vi "Andres  Decoder 3-to-4 while-loop (why run only once).vi"() -> ()   [LabVIEW 2013]
panel:
  out "Boolean 4":bool
  out "Boolean 3":bool
  out "Boolean 2":bool
  out "Boolean 1":bool
  out "Boolean 0":bool
  in  "Digital 2":bool
  in  "Digital 0":bool
  in  "Digital 1":bool
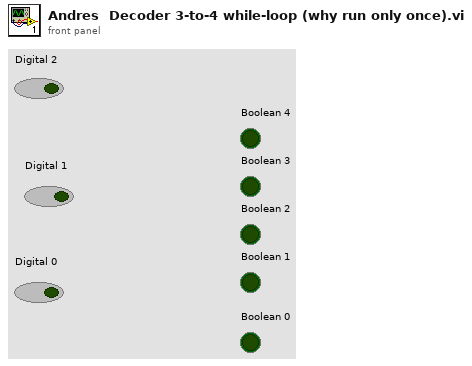
[diagram p1: front panel]
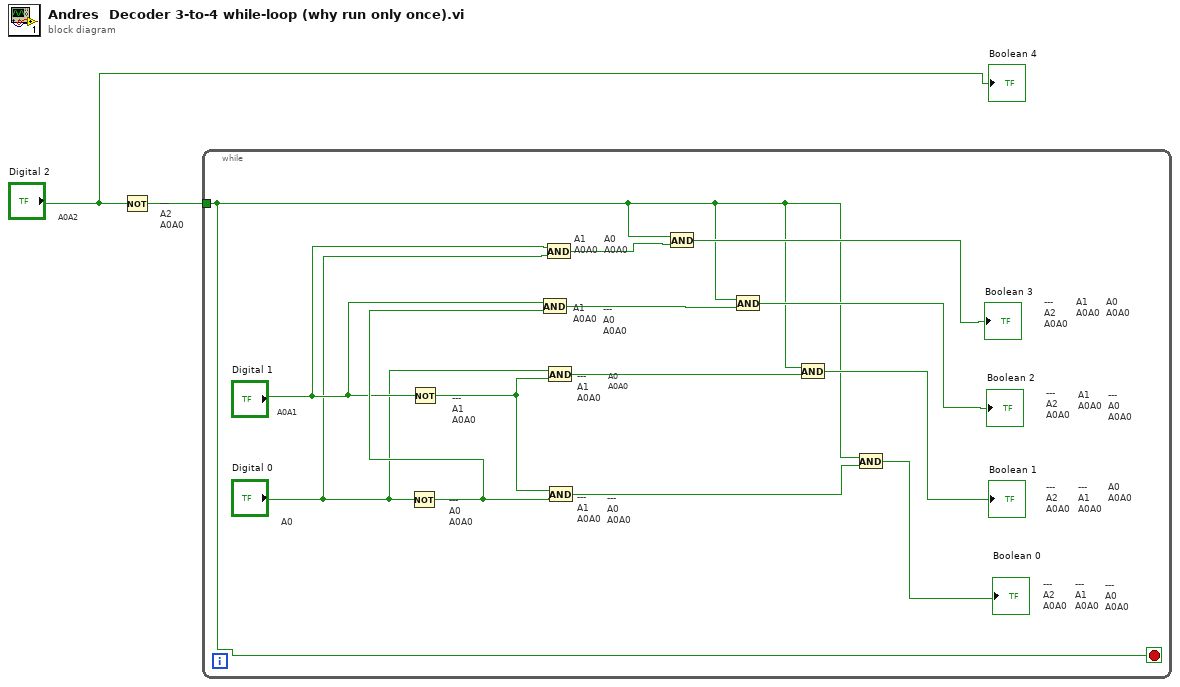
[diagram p0: block diagram]
diagram:
  # "---\nA2\nA0A0"
  # "A0A2"
  n1 = Not(x="Digital 2") -> (.not. x?=w2:bool)
  n2 = while {
    tunnel: w2 -> [w3]
    stop <- w3 stop-if-true
    # "A1\nA0A0"
    # "A0\nA0A0"
    # "---\nA2\nA0A0"
    # "A1\nA0A0"
    # "A0\nA0A0"
    # "A1\nA0A0"
    # "---\nA0\nA0A0"
    # "---\nA2\nA0A0"
    # "A1\nA0A0"
    # "---\nA0\nA0A0"
    # "---\nA1\nA0A0"
    # "A0\nA0A0"
    # "---\nA2\nA0A0"
    # "---\nA1\nA0A0"
    # "A0\nA0A0"
    # "---\nA2\nA0A0"
    # "---\nA1\nA0A0"
    # "---\nA0\nA0A0"
    # "---\nA1\nA0A0"
    # "---\nA0\nA0A0"
    # "---\nA1\nA0A0"
    # "A0A1"
    # "---\nA0\nA0A0"
    # "A0"
    n3 = Not(x="Digital 0") -> (.not. x?=w10:bool)
    n4 = Not(x="Digital 1") -> (.not. x?=w13:bool)
    n5 = And(x="Digital 1", y=w10) -> (x .and. y?=w9:bool)
    n6 = And(x="Digital 1", y="Digital 0") -> (x .and. y?=w5:bool)
    n7 = And(x="Digital 0", y=w13) -> (x .and. y?=w12:bool)
    n8 = And(x=w13, y=w10) -> (x .and. y?=w15:bool)
    n9 = And(x=w3, y=w5) -> (x .and. y?=→"Boolean 3":bool)
    n10 = And(x=w3, y=w9) -> (x .and. y?=→"Boolean 2":bool)
    n11 = And(x=w3, y=w12) -> (x .and. y?=→"Boolean 1":bool)
    n12 = And(x=w3, y=w15) -> (x .and. y?=→"Boolean 0":bool)
  }
  "Boolean 4" <- "Digital 2"
